vi "plot.issues.vi"(5 "volume.volume type":T1 caption="Enum", 6 "in collections":bool[](array[boolean]), 7 "volume_name":string, 8 "error in (no error)":errorcluster, 9 "cover_dates":timestamp[](array[timestamp]), 10 "issue_numbers":string[](array[string]), 11 "picture ref":refnum<vi>) -> (0 "error out":errorcluster, 3 "reference out":refnum<vi>)   [LabVIEW 2024]
uses:
  Graphic_UI/typedefs/volume.type.colors--cluster.ctl
  CV_Shared_Library/volume.type--enum.ctl
  CV_Shared_Library/CV_Shared_Library.lvlib
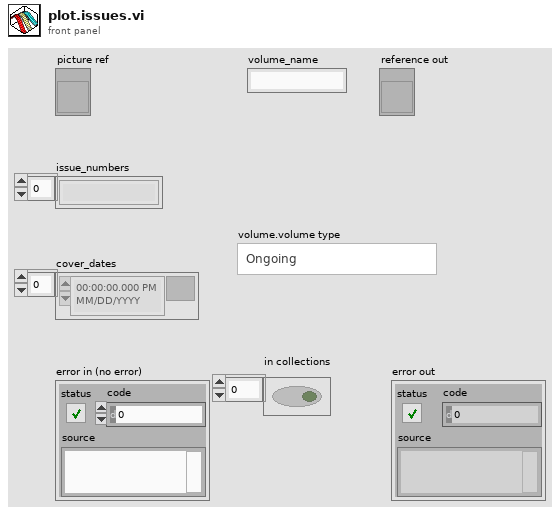
[diagram p1: front panel]
types:
  T1 = typedef "CV_Shared_Library.lvlib/volume.type--enum.ctl" = enum16{"Ongoing", "Limited Series", "Annual", "One Shot", "Reprint/Document", "Digital"}
  T2 = cluster{"Width":u16, "Style":enum32{"Solid", "Dash", "Dot", "DashDot", "DashDotDot"}}
  T3 = typedef "volume.type.colors--cluster.ctl" = cluster{"ongoing":u32, "Limited Series":u32, "Annuals":u32, "One Shots":u32, "Reprints":u32, "Digital":u32}
  T4 = cluster{"left":i16, "top":i16, "right":i16, "bottom":i16}
  T5 = cluster{"Time Stamp":timestamp, "String":string}[]
  T6 = typedef "LVBoundsTypeDef.ctl" = cluster{"Width":u32, "Height":u32}
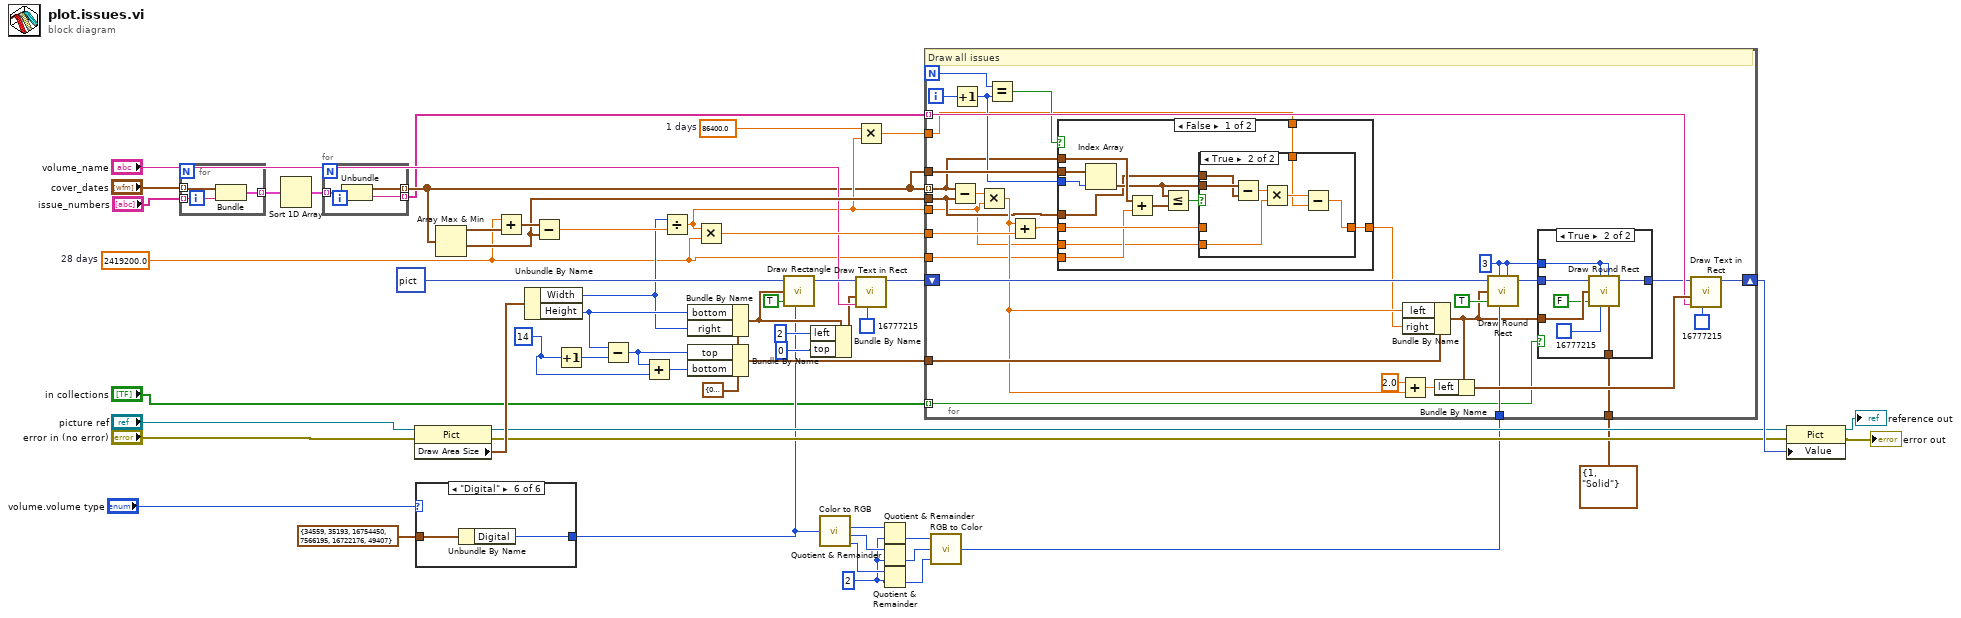
[diagram p0: block diagram]
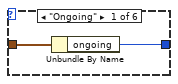
[diagram p2: hidden frame]
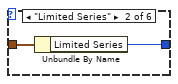
[diagram p3: hidden frame]
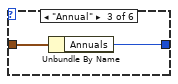
[diagram p4: hidden frame]
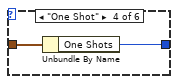
[diagram p5: hidden frame]
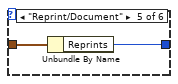
[diagram p6: hidden frame]
diagram:
  w12 = 86400.0  # 1 days
  w17 = u8 2 ("y")
  w39 = i16 14 ("y")
  w33 = T4 {"left"=0, "top"=0, "right"=0, "bottom"=0} ("rect")
  w9 = 2419200.0  # 28 days
  n1 = for {
    tunnel: "issue_numbers" -> [w57] mode=indexing
    tunnel: "cover_dates" -> [w56] mode=indexing
    tunnel: [w55] -> w8 mode=indexing
    n2 = Bundle("Time Stamp"=w56, "String"=w57) -> (w55:cluster{"Time Stamp":timestamp, "String":string})  [unwired: 1 in]
  }
  n3 = Sort 1D Array(array=w8) -> (sorted array=w7:T5)
  n4 = for {
    tunnel: w7 -> [w60] mode=indexing
    tunnel: [w59] -> w5 mode=indexing
    tunnel: [w58] -> w3 mode=indexing
    n5 = Unbundle(w60) -> ("Time Stamp"=w59:timestamp, "String"=w58:string)
  }
  n6 = property class="Pict"(reference="picture ref", error in="error in (no error)") -> (reference out=w45:refnum<vi>, error out=w44:errorcluster, "Draw Area Size"=w50:T6)
  n7 = case shown="\"Digital\"" "volume.volume type" {
    tunnel: T3 {"ongoing"=34559, "Limited Series"=35193, "Annuals"=16754450, "One Shots"=7566195, "Reprints"=16722176, "Digital"=49407} ("Legend") -> [w62 w64 w66 w68 w70 w72]
    tunnel: [w61 w63 w65 w67 w69 w71] -> w21
    frame "Ongoing" {
      n8 = Unbundle By Name(w62) -> ("ongoing"=w61:u32)
    }
    frame "Limited Series" {
      n9 = Unbundle By Name(w64) -> ("Limited Series"=w63:u32)
    }
    frame "Annual" {
      n10 = Unbundle By Name(w66) -> ("Annuals"=w65:u32)
    }
    frame "One Shot" {
      n11 = Unbundle By Name(w68) -> ("One Shots"=w67:u32)
    }
    frame "Reprint/Document" {
      n12 = Unbundle By Name(w70) -> ("Reprints"=w69:u32)
    }
    frame "Digital" {
      n13 = Unbundle By Name(w72) -> ("Digital"=w71:u32)
    }
  }
  n14 = Array Max & Min(array=w5) -> (max value=w52:timestamp, min value=w48:timestamp)  [unwired: 2 out]
  n15 = Add(x=w9, y=w52) -> (x+y=w51:timestamp)
  n16 = Unbundle By Name(w50) -> ("Width"=w31:u32, "Height"=w32:u32)
  n17 = Subtract(x=w51, y=w48) -> (x-y=w49:dbl)
  n18 = Increment(x=w39) -> (x+1=w41:i16)
  n19 = Subtract(x=w32, y=w41) -> (x-y=w40:u32)
  n20 = Add(x=w40, y=w39) -> (x+y=w38:u32)
  n21 = Divide(x=w31, y=w49) -> (x/y=w11:dbl)
  n22 = Bundle By Name(cluster=w33, "bottom"=w32, "right"=w31) -> (w25:T4)
  n23 = Bundle By Name(cluster=w33, "top"=w40, "bottom"=w38) -> (w34:T4)
  n24 = Multiply(x=w11, y=w9) -> (x*y=w47:dbl)
  n25 = call <vilib>:"Draw Rectangle.vi"("picture"=picture data[5B], "rect"=w25, "fill?(F)"=TRUE, "color(black)"=w21) -> ("new picture"=w29:picture)  [unwired: 5 in]
  n26 = Bundle By Name(cluster=w25, "left"=i16 2, "top"=i16 0) -> (w26:T4)
  n27 = call <vilib>:"Color to RGB.vi"("Color"=w21) -> ("R"=w20:u8, "G"=w19:u8, "B"=w18:u8)  [unwired: 1 out]
  n28 = Multiply(x=w12, y=w11) -> (x*y=w10:dbl)
  n29 = call <vilib>:"Draw Text in Rect.vi"("text color(black)"=u32 16777215, "text"="volume_name", "rect"=w26, "picture"=w29) -> ("new picture"=w28:picture)  [unwired: 7 in]
  n30 = Quotient & Remainder(x=w20, y=w17) -> (floor(x/y)=w16:u8)  [unwired: 1 out]
  n31 = Quotient & Remainder(x=w19, y=w17) -> (floor(x/y)=w15:u8)  [unwired: 1 out]
  n32 = Quotient & Remainder(x=w18, y=w17) -> (floor(x/y)=w14:u8)  [unwired: 1 out]
  n33 = call <vilib>:"RGB to Color.vi"("B"=w14, "G"=w15, "R"=w16) -> ("Color"=w13:u32)
  n34 = for {
    N -> [w89]
    tunnel: w11 -> [w80]
    tunnel: w48 -> [w81]
    tunnel: w47 -> [w102]
    tunnel: w34 -> [w101]
    shift-right: [w95] -> w46
    shift-left: w28 -> [w100]
    tunnel: w3 -> [w92] mode=indexing
    tunnel: w5 -> [w82] mode=indexing
    tunnel: w13 -> [w91]
    tunnel: w5 -> [w85]
    tunnel: w10 -> [w79]
    tunnel: w9 -> [w83]
    tunnel: "in collections" -> [w78] mode=indexing
    tunnel: T2 {"Width"=1, "Style"=enum."Solid"} ("pen") -> [w73]
    i -> [w90]
    w77 = i16 3 ("oval width")
    # "Draw all issues"
    n35 = Subtract(x=w82, y=w81) -> (x-y=w103:dbl)
    n36 = Increment(x=w90) -> (x+1=w84:i32)
    n37 = Multiply(x=w103, y=w80) -> (x*y=w99:dbl)
    n38 = Equal?(x=w89, y=w84) -> (x = y?=w88:bool)
    n39 = Add(x=w99, y=w102) -> (x+y=w86:dbl)
    n40 = case shown="False" w88 {
      tunnel: [w120 w132] -> w87
      tunnel: w86 -> [w119 w132]
      tunnel: w85 -> [w123 _]
      tunnel: w84 -> [w122 _]
      tunnel: w83 -> [w118 _]
      tunnel: w82 -> [w116 _]
      tunnel: w81 -> [w114 _]
      tunnel: w80 -> [w113 _]
      tunnel: w79 -> [w112 _]
      frame False {
        n41 = Index Array(array=w123, index=w122) -> (element=w115:timestamp)
        n42 = Add(x=w116, y=w118) -> (x+y=w117:timestamp)
        n43 = Less Or Equal?(x=w115, y=w117) -> (x <= y?=w121:bool)
        n44 = case shown="True" w121 {
          tunnel: [w124 w125] -> w120
          tunnel: w119 -> [w124 _]
          tunnel: w115 -> [_ w131]
          tunnel: w114 -> [_ w130]
          tunnel: w113 -> [_ w128]
          tunnel: w112 -> [_ w126]
          frame False {
          }
          frame True {
            n45 = Subtract(x=w131, y=w130) -> (x-y=w129:dbl)
            n46 = Multiply(x=w129, y=w128) -> (x*y=w127:dbl)
            n47 = Subtract(x=w127, y=w126) -> (x-y=w125:dbl)
          }
        }
      }
      frame True {
      }
    }
    n48 = Add(x=2.0, y=w99) -> (x+y=w97:dbl)
    n49 = Bundle By Name(cluster=w101, "left"=w99, "right"=w87) -> (w74:T4)
    n50 = Bundle By Name(cluster=w74, "left"=w97) -> (w94:T4)
    n51 = call <vilib>:"Draw Round Rect.vi"("picture"=w100, "oval width"=w77, "rect"=w74, "fill?(F)"=TRUE, "color(black)"=w91, "oval height"=w77) -> ("new picture"=w76:picture)  [unwired: 3 in]
    n52 = case shown="True" w78 {
      tunnel: w77 -> [_ w111]
      tunnel: w76 -> [w104 w110]
      tunnel: [w104 w109] -> w75
      tunnel: w74 -> [_ w108]
      tunnel: w73 -> [_ w105]
      frame False {
      }
      frame True {
        n53 = call <vilib>:"Draw Round Rect.vi"("picture"=w110, "oval width"=w111, "rect"=w108, "fill?(F)"=FALSE, "color(black)"=u32 16777215, "oval height"=w111, "pen"=w105) -> ("new picture"=w109:picture)  [unwired: 2 in]
      }
    }
    n54 = call <vilib>:"Draw Text in Rect.vi"("text color(black)"=u32 16777215, "text"=w92, "rect"=w94, "picture"=w75) -> ("new picture"=w95:picture)  [unwired: 7 in]
  }
  n55 = property class="Pict"(reference=w45, error in=w44, "Value"=w46) -> (reference out=→"reference out":refnum<vi>, error out=→"error out":errorcluster)
